vi "obj_DataLog Table Columns.vi"(0 "method":T7, 7 "tag":string, 9 "index":i32, 11 "error in (no error)":errorcluster, 12 "database":string, 13 "database infos":T8, 14 "table ref":refnum<vi>) -> (3 "column index":i32, 4 "#columns":i32, 6 "flag":bool, 8 "tag config":T2 {"logging parameters" format="%.2e"; "precision" items=["0", "1", "2", "3", "4", "5", "6", "7", "8", "9", "10", "11", "12", "13", "14", "15", "16", "17"]; "limit delay" format="%.2e"; "deadband" format="%.2e"}, 10 "mode":T1, 15 "error out":errorcluster)   [LabVIEW 2012]
doc: "Manages the addition, display, sorting, reordering, deletion, etc. of tags to/from the columns of the table control of the \"Log Table\" GUI."
uses:
  typedefs/t_Datalog Table Columns Methods.ctl
  typedefs/clusters/t_DataLog Tag Config.ctl
  typedefs/t_DataLog Temporal Types.ctl
  typedefs/t_DataLog Value Types.ctl
  typedefs/t_DataLog Numerical Format.ctl
  typedefs/t_DataLog Logging Algorithms.ctl
  typedefs/t_DataLog Table Retrieval Modes.ctl
  served/DataLog Database Infos_srv.ctl
  typedefs/t_DataLog Tag Info List Methods.ctl
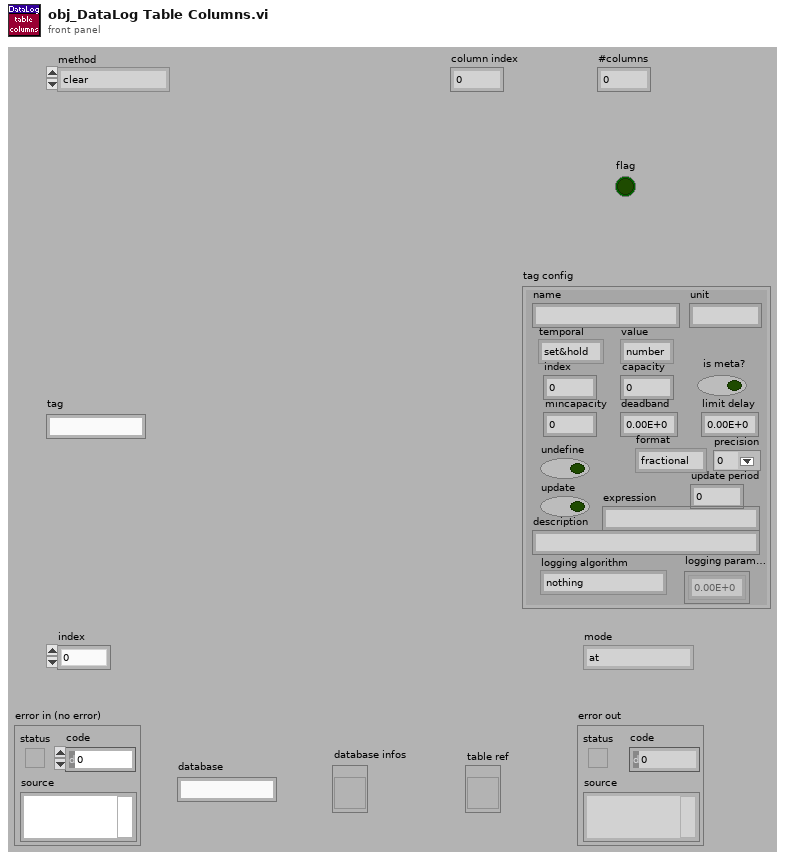
[diagram p1: front panel]
types:
  T1 = typedef "t_DataLog Table Retrieval Modes.ctl" = enum16{"at", "interpolate", "at+interpolate"}
  T2 = typedef "t_DataLog Tag Config.ctl" = cluster{"name":string, "unit":string, "temporal":T3, "value":T4, "index":i32, "capacity":i32, "is meta?":bool, "mincapacity":i32, "deadband":dbl, "limit delay":dbl, "format":T5, "precision":u8, "undefine":bool, "update":bool, "update period":u16, "expression":string, "description":string, "logging algorithm":T6, "logging parameters":dbl[]}
  T3 = typedef "t_DataLog Temporal Types.ctl" = enum16{"set&hold", "sample", "event"}
  T4 = typedef "t_DataLog Value Types.ctl" = enum16{"number", "string"}
  T5 = typedef "t_DataLog Numerical Format.ctl" = enum8{"fractional", "exponential", "engineering"}
  T6 = typedef "t_DataLog Logging Algorithms.ctl" = enum16{"nothing", "changes", "everything", "every Nth", "time threshold", "value threshold + prior", "t or v threshold", "t or v threshold + prior"}
  T7 = typedef "t_Datalog Table Columns Methods.ctl" = enum16{"clear", "#columns", "#number", "add", "insert", "remove", "change mode", "reorder", "sort", "index", "get by name", "interpolatable?", "ats?", "update"}
  T8 = typedef "DataLog Database Infos_srv.ctl" = refnum<vi>
  T9 = typedef "t_DataLog Tag Info List Methods.ctl" = enum16{"initialize", "create", "create empty", "rename", "delete", "test tag", "get", "get by name", "get default", "get list", "get path", "get subsets", "set subsets", "set config", "set capacity", "#tags", "go live", "set unlocked", "set mirrored"}
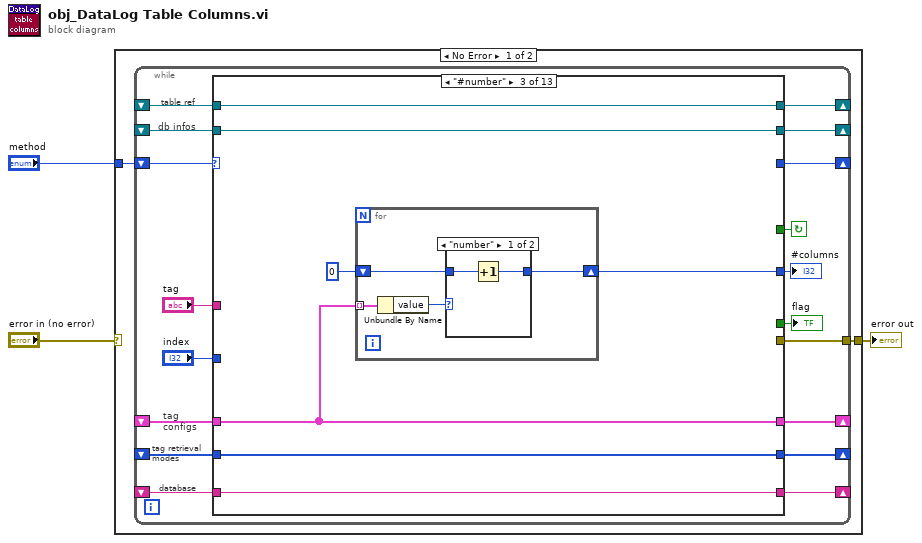
[diagram p0: block diagram]
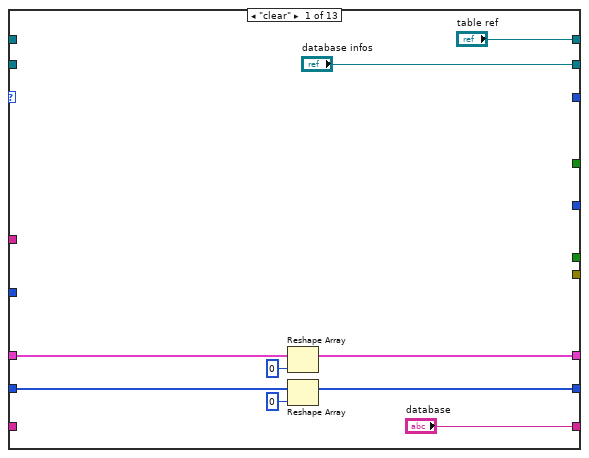
[diagram p2: hidden frame]
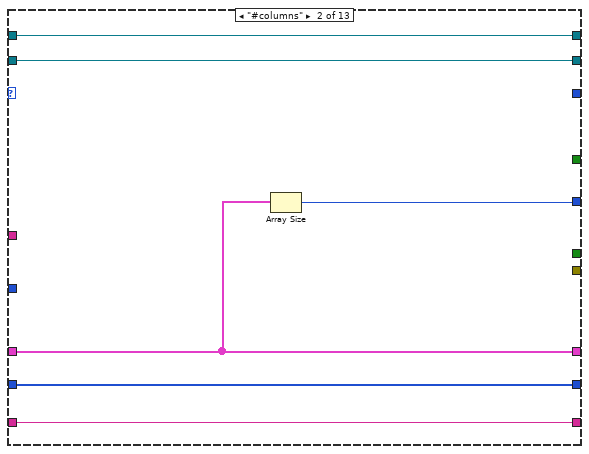
[diagram p3: hidden frame]
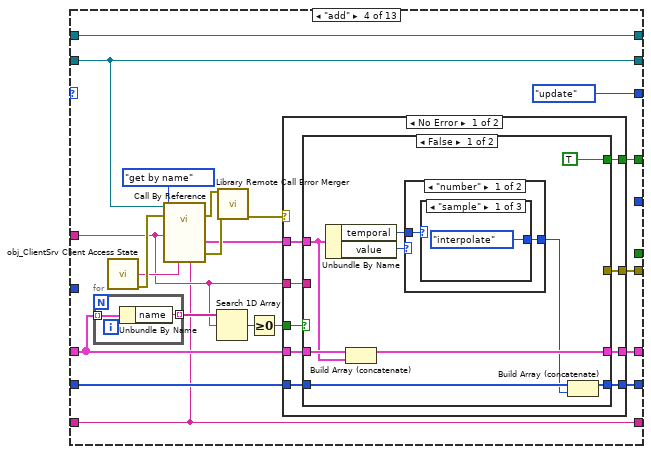
[diagram p5: hidden frame]
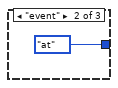
[diagram p6: hidden frame]
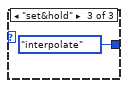
[diagram p7: hidden frame]
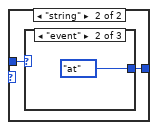
[diagram p8: hidden frame]
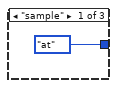
[diagram p9: hidden frame]
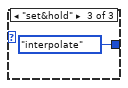
[diagram p10: hidden frame]
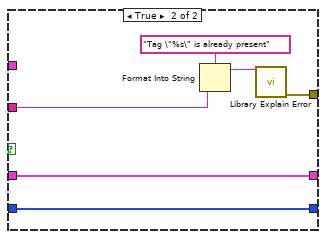
[diagram p11: hidden frame]
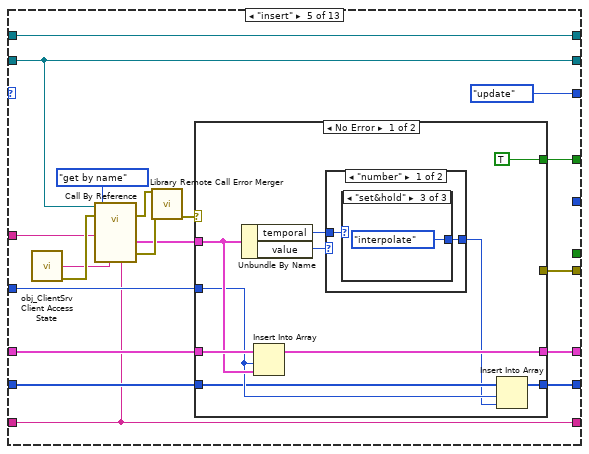
[diagram p13: hidden frame]
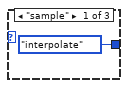
[diagram p14: hidden frame]
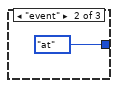
[diagram p15: hidden frame]
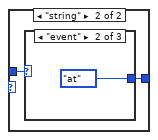
[diagram p16: hidden frame]
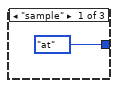
[diagram p17: hidden frame]
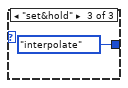
[diagram p18: hidden frame]
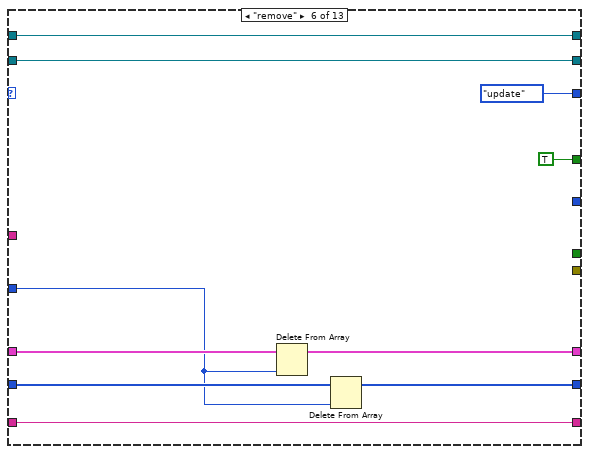
[diagram p20: hidden frame]
diagram:
  n1 = case shown="No Error" "error in (no error)" {
    selector: "error in (no error)" -> [_ w313]
    tunnel: [w4 w313] -> w2
    tunnel: "method" -> [w5 _]
    frame No Error {
      n2 = while {
        shift-right: [w23] -> _
        shift-left: _ -> [w22]
        shift-right: [w21] -> _
        shift-left: _ -> [w20]
        shift-right: [w19] -> _
        shift-left: _ -> [w18]
        shift-right: [w14] -> _
        shift-left: _ -> [w17]
        shift-right: [w15] -> _
        shift-left: _ -> [w16]
        shift-right: [w12] -> _
        shift-left: w5 -> [w13]
        tunnel: [w9] -> w4
        stop <- w11 continue-if-true
        # "tag retrieval\nmodes"
        # "tag\nconfigs"
        # "db infos"
        # "table ref"
        # "database"
        n3 = case shown="\"#number\"" w13 {
          selector: w13 -> [_ _ _ _ _ _ _ _ _ w232 _ _ _]
          tunnel: ["database infos" w36 w43 w59 w115 w162 w173 w190 w218 w237 w255 w278 w291] -> w23
          tunnel: w22 -> [_ w36 w43 w59 w115 w162 w173 w190 w218 w237 w255 w278 w291]
          tunnel: ["database" w37 w44 w53 w113 w164 w175 w191 w219 w238 w256 w279 w293] -> w21
          tunnel: w20 -> [_ w37 w44 w53 w113 w164 w175 w191 w219 w238 w256 w279 w293]
          tunnel: ["table ref" w35 w42 w73 w131 w163 w174 w189 w217 w236 w254 w277 w288] -> w19
          tunnel: w18 -> [_ w35 w42 w73 w131 w163 w174 w189 w217 w236 w254 w277 w288]
          tunnel: w17 -> [w29 w34 w41 w58 w123 w159 w170 w183 w213 w228 w252 w276 w292]
          tunnel: w16 -> [w26 w38 w45 w64 w120 w157 w168 w180 w220 w233 w253 w273 w294]
          tunnel: [w24 w38 w45 w63 w119 w156 w167 w181 w220 w233 w253 w273 w294] -> w15
          tunnel: [w27 w34 w41 w66 w122 w158 w170 w182 w212 w227 w252 w276 w292] -> w14
          tunnel: [_ _ _ t_Datalog_Table_Columns_Methods."update" ("method") t_Datalog_Table_Columns_Methods."update" ("method") t_Datalog_Table_Columns_Methods."update" ("method") t_Datalog_Table_Columns_Methods."update" ("method") t_Datalog_Table_Columns_Methods."update" ("method") t_Datalog_Table_Columns_Methods."update" ("method") _ _ _ _] -> w12
          tunnel: [_ _ _ w60 w116 TRUE TRUE w188 TRUE _ _ _ _] -> w11
          tunnel: "tag" -> [_ _ _ w54 w124 _ _ _ _ w231 _ _ _]
          tunnel: [_ _ _ w61 w117 _ _ _ _ _ _ _ w289] -> w9
          tunnel: "index" -> [_ _ _ _ w114 w155 w166 _ _ w230 w251 _ _]
          tunnel: [_ _ _ _ _ _ _ _ _ _ w249 w274 _] -> w7
          tunnel: [_ w33 w39 _ _ _ _ _ _ _ _ _ _] -> w6
          frame "clear" {
            n4 = Reshape Array(w29, 0 ("dimension size")) -> (w27:T2[])
            n5 = Reshape Array(w26, 0 ("dimension size")) -> (w24:T1[])
          }
          frame "#columns" {
            n6 = Array Size(array=w34) -> (size(s)=w33:i32)
          }
          frame "#number" {
            n7 = for {
              tunnel: w41 -> [w49] mode=indexing
              shift-right: [w47] -> w39
              shift-left: 0 -> [w46]
              n8 = Unbundle By Name(w49) -> ("value"=w48:T4)
              n9 = case shown="\"number\"" w48 {
                tunnel: [w51 w52] -> w47
                tunnel: w46 -> [w50 w52]
                frame "number" {
                  n10 = Increment(x=w50) -> (x+1=w51:i32)
                }
                frame "string" {
                }
              }
            }
          }
          frame "add" {
            n11 = for {
              tunnel: w58 -> [w75] mode=indexing
              tunnel: [w74] -> w57 mode=indexing
              n12 = Unbundle By Name(w75) -> ("name"=w74:string)
            }
            n13 = call "obj_ClientSrv Client Access State.vi"() -> ("certificate"=w69:string, "error out"=w71:errorcluster)  [unwired: 14 in]
            n14 = call-by-ref "?"(reference=w59, error in=w71, "method"=t_DataLog_Tag_Info_List_Methods."get by name", "tag or base tag"=w54, "certificate in"=w69, "database (current)"=w53) -> (error out=w72:errorcluster, "tag config out"=w65:T2, 15:"error out"=w70:errorcluster)  [unwired: 6 in, 5 out]
            n15 = Search 1D Array(1D array=w57, element=w54) -> (index of element=w56:i32)  [unwired: 1 in]
            n16 = call "Library Remote Call Error Merger.vi"("call by reference node error"=w72, "called VI error (no error)"=w70) -> ("error out"=w62:errorcluster)  [unwired: 13 in]
            n17 = Greater Or Equal To 0?(x=w56) -> (x >= 0?=w55:bool)
            n18 = case shown="No Error" w62 {
              selector: w62 -> [_ w112]
              tunnel: w58 -> [w84 w111]
              tunnel: [w83 w111] -> w66
              tunnel: w65 -> [w82 _]
              tunnel: w64 -> [w81 w110]
              tunnel: [w80 w110] -> w63
              tunnel: [w76 w112] -> w61
              tunnel: [w79 _] -> w60
              tunnel: w55 -> [w78 _]
              tunnel: w54 -> [w77 _]
              frame No Error {
                n19 = case shown="False" w78 {
                  tunnel: w84 -> [w93 w109]
                  tunnel: [w92 w109] -> w83
                  tunnel: w82 -> [w91 _]
                  tunnel: w81 -> [w88 w108]
                  tunnel: [w87 w108] -> w80
                  tunnel: [TRUE _] -> w79
                  tunnel: w77 -> [_ w104]
                  tunnel: [_ w107] -> w76
                  frame False {
                    n20 = Unbundle By Name(w91) -> ("temporal"=w90:T3, "value"=w89:T4)
                    n21 = Build Array (concatenate)(w93, w91) -> (w92:T2[])
                    n22 = case shown="\"number\"" w89 {
                      tunnel: w90 -> [w95 w100]
                      tunnel: [w94 w99] -> w86
                      frame "number" {
                        n23 = case shown="\"sample\"" w95 {
                          tunnel: [t_DataLog_Table_Retrieval_Modes."interpolate" ("retrieval modes") t_DataLog_Table_Retrieval_Modes."at" ("retrieval modes") t_DataLog_Table_Retrieval_Modes."interpolate" ("retrieval modes")] -> w94
                          frame "sample" {
                          }
                          frame "event" {
                          }
                          frame "set&hold" {
                          }
                        }
                      }
                      frame "string" {
                        n24 = case shown="\"event\"" w100 {
                          tunnel: [t_DataLog_Table_Retrieval_Modes."at" ("retrieval modes") t_DataLog_Table_Retrieval_Modes."at" ("retrieval modes") t_DataLog_Table_Retrieval_Modes."interpolate" ("retrieval modes")] -> w99
                          frame "sample" {
                          }
                          frame "event" {
                          }
                          frame "set&hold" {
                          }
                        }
                      }
                    }
                    n25 = Build Array (concatenate)(w88, w86) -> (w87:T1[])
                  }
                  frame True {
                    n26 = Format Into String(format string="Tag \"%s\" is already present", w104) -> (resulting string=w106:string)  [unwired: 2 in, 1 out]
                    n27 = call "Library Explain Error.vi"("explanation prefix (none)"=w106) -> ("explained error"=w107:errorcluster)  [unwired: 14 in]
                  }
                }
              }
              frame Error {
              }
            }
          }
          frame "insert" {
            n28 = call "obj_ClientSrv Client Access State.vi"() -> ("certificate"=w127:string, "error out"=w129:errorcluster)  [unwired: 14 in]
            n29 = call-by-ref "?"(reference=w115, error in=w129, "method"=t_DataLog_Tag_Info_List_Methods."get by name", "tag or base tag"=w124, "certificate in"=w127, "database (current)"=w113) -> (error out=w130:errorcluster, "tag config out"=w121:T2, 15:"error out"=w128:errorcluster)  [unwired: 6 in, 5 out]
            n30 = call "Library Remote Call Error Merger.vi"("call by reference node error"=w130, "called VI error (no error)"=w128) -> ("error out"=w118:errorcluster)  [unwired: 13 in]
            n31 = case shown="No Error" w118 {
              selector: w118 -> [_ w154]
              tunnel: w123 -> [w141 w153]
              tunnel: [w140 w153] -> w122
              tunnel: w121 -> [w136 _]
              tunnel: w120 -> [w134 w152]
              tunnel: [w133 w152] -> w119
              tunnel: [_ w154] -> w117
              tunnel: [TRUE _] -> w116
              tunnel: w114 -> [w135 _]
              frame No Error {
                n32 = Unbundle By Name(w136) -> ("temporal"=w139:T3, "value"=w138:T4)
                n33 = Insert Into Array(array=w141, index=w135, new element=w136) -> (w140:T2[])
                n34 = case shown="\"number\"" w138 {
                  tunnel: w139 -> [w143 w148]
                  tunnel: [w142 w147] -> w132
                  frame "number" {
                    n35 = case shown="\"set&hold\"" w143 {
                      tunnel: [t_DataLog_Table_Retrieval_Modes."interpolate" ("retrieval modes") t_DataLog_Table_Retrieval_Modes."at" ("retrieval modes") t_DataLog_Table_Retrieval_Modes."interpolate" ("retrieval modes")] -> w142
                      frame "sample" {
                      }
                      frame "event" {
                      }
                      frame "set&hold" {
                      }
                    }
                  }
                  frame "string" {
                    n36 = case shown="\"event\"" w148 {
                      tunnel: [t_DataLog_Table_Retrieval_Modes."at" ("retrieval modes") t_DataLog_Table_Retrieval_Modes."at" ("retrieval modes") t_DataLog_Table_Retrieval_Modes."interpolate" ("retrieval modes")] -> w147
                      frame "sample" {
                      }
                      frame "event" {
                      }
                      frame "set&hold" {
                      }
                    }
                  }
                }
                n37 = Insert Into Array(array=w134, index=w135, new element=w132) -> (w133:T1[])
              }
              frame Error {
              }
            }
          }
          frame "remove" {
            n38 = Delete From Array(array=w159, index=w155) -> (array with subset deleted=w158:T2[])  [unwired: 1 in, 1 out]
            n39 = Delete From Array(array=w157, index=w155) -> (array with subset deleted=w156:T1[])  [unwired: 1 in, 1 out]
          }
          frame "change mode" {
            n40 = Index Array(array=w168, index=w166) -> (element=w169:T1)
            n41 = case shown="\"at\"" w169 {
              tunnel: [t_DataLog_Table_Retrieval_Modes."at+interpolate" ("retrieval modes") t_DataLog_Table_Retrieval_Modes."at" ("retrieval modes") t_DataLog_Table_Retrieval_Modes."interpolate" ("retrieval modes")] -> w165
              frame "interpolate" {
              }
              frame "at+interpolate" {
              }
              frame "at" {
              }
            }
            n42 = Replace Array Subset(array=w168, new element=w165, index=w166) -> (w167:T1[])
          }
          frame "reorder" {
            n43 = for {
              tunnel: w183 -> [w209] mode=indexing
              tunnel: [w208] -> w184 mode=indexing
              n44 = Unbundle By Name(w209) -> ("name"=w208:string)
            }
            n45 = call "ui_DataLog Reorder Listed Strings.vi"("prompt"="Reorder tag columns:", "list of strings"=w184) -> ("OKed?"=w186:bool, "reordered strings"=w185:string[])  [unwired: 12 in]
            n46 = case shown="True" w186 {
              tunnel: [_ TRUE] -> w188
              tunnel: w185 -> [_ w199]
              tunnel: w184 -> [_ w198]
              tunnel: w183 -> [w193 w197]
              tunnel: [w193 w196] -> w182
              tunnel: [w192 w195] -> w181
              tunnel: w180 -> [w192 w194]
              frame False {
              }
              frame True {
                n47 = for {
                  tunnel: w199 -> [w206] mode=indexing
                  tunnel: w198 -> [w207]
                  tunnel: w197 -> [w205]
                  tunnel: [w204] -> w196 mode=indexing
                  tunnel: [w203] -> w195 mode=indexing
                  tunnel: w194 -> [w202]
                  n48 = Search 1D Array(1D array=w207, element=w206) -> (index of element=w201:i32)  [unwired: 1 in]
                  n49 = Index Array(array=w205, index=w201) -> (element=w204:T2)
                  n50 = Index Array(array=w202, index=w201) -> (element=w203:T1)
                }
              }
            }
          }
          frame "sort" {
            # "avoid LV7 bug"
            n51 = for "prepend for sorting" {
              tunnel: w213 -> [w224] mode=indexing
              tunnel: [w226] -> w215 mode=indexing
              # "Lower case. This makes\nthe sort case insensitive\nand gives the underscore\na lower priority so that\nmeta tags group with\ntheir base tag."
              n52 = Unbundle By Name(w224) -> ("name"=w223:string)
              n53 = To Lower Case(string=w223) -> (all lower case string=w225:string)
              n54 = Bundle(w225, "tag config out"=w224) -> (w226:cluster{string, "tag config out":T2})  [unwired: 1 in]
            }
            n55 = Sort 1D Array(array=w215) -> (sorted array=w216:cluster{string, "tag config out":T2}[])
            n56 = Sort 1D Array(array=w216) -> (sorted array=w214:cluster{string, "tag config out":T2}[])
            n57 = for {
              tunnel: w214 -> [w222] mode=indexing
              tunnel: [w221] -> w212 mode=indexing
              n58 = Unbundle(w222) -> ("tag config out"=w221:T2)  [unwired: 1 out]
            }
          }
          frame "index", "get by name" {
            n59 = case shown="\"get by name\"" w232 {
              tunnel: w231 -> [_ _ w244]
              tunnel: w230 -> [w240 w242 _]
              tunnel: [w240 w242 w243] -> w229
              tunnel: w228 -> [w239 w241 w246]
              tunnel: [w239 w241 w246] -> w227
              frame Default {
              }
              frame "index" {
              }
              frame "get by name" {
                n60 = for {
                  tunnel: w246 -> [w248] mode=indexing
                  tunnel: [w247] -> w245 mode=indexing
                  n61 = Unbundle By Name(w248) -> ("name"=w247:string)
                }
                n62 = Search 1D Array(1D array=w245, element=w244) -> (index of element=w243:i32)  [unwired: 1 in]
                "column index" <- w243
              }
            }
            n63 = Index Array(array=w227, index=w229) -> (element=→"tag config":T2)
            n64 = Index Array(array=w233, index=w229) -> (element=→"mode":T1)
          }
          frame "interpolatable?" {
            n65 = Greater Or Equal To 0?(x=w251) -> (x >= 0?=w250:bool)
            n66 = case shown="True" w250 {
              tunnel: w252 -> [_ w259]
              tunnel: [_ w258] -> w249
              tunnel: w251 -> [_ w257]
              frame False {
              }
              frame True {
                n67 = Index Array(array=w259, index=w257) -> (element=w260:T2)
                n68 = Unbundle By Name(w260) -> ("temporal"=w262:T3, "value"=w261:T4)
                n69 = case shown="\"number\"" w261 {
                  tunnel: w262 -> [w264 w269]
                  tunnel: [w263 w268] -> w258
                  frame "number" {
                    n70 = case shown="\"set&hold\"" w264 {
                      tunnel: [TRUE FALSE TRUE] -> w263
                      frame "sample" {
                      }
                      frame "event" {
                      }
                      frame "set&hold" {
                      }
                    }
                  }
                  frame "string" {
                    n71 = case shown="\"event\"" w269 {
                      tunnel: [FALSE FALSE TRUE] -> w268
                      frame "sample" {
                      }
                      frame "event" {
                      }
                      frame "set&hold" {
                      }
                    }
                  }
                }
              }
            }
          }
          frame "ats?" {
            n72 = for {
              shift-right: [w280] -> w274
              shift-left: FALSE -> [w281]
              tunnel: w273 -> [w282] mode=indexing
              n73 = case shown="\"at\", \"at+interpolate\"" w282 {
                tunnel: w281 -> [_ w284]
                tunnel: [TRUE w284] -> w280
                frame "at", "at+interpolate" {
                }
                frame "interpolate" {
                }
              }
            }
          }
          frame "update" {
            n74 = for {
              tunnel: w292 -> [w311] mode=indexing
              tunnel: [w308] -> w290 mode=indexing
              tunnel: w294 -> [w307] mode=indexing
              tunnel: [" "] -> w287 mode=indexing
              w312 = "\n"
              n75 = Unbundle By Name(w311) -> ("temporal"=w305:T3, "value"=w304:T4, "name"=w310:string, "unit"=w309:string, "logging algorithm"=w300:T6)
              n76 = Format Into String(w307) -> (resulting string=w303:string)  [unwired: 3 in, 1 out]
              n77 = Equal?(x=w300, y=t_DataLog_Logging_Algorithms."nothing" ("logging algorithm")) -> (x = y?=w298:bool)
              n78 = Format Into String(format string="%s/%s", w305, w304) -> (resulting string=w302:string)  [unwired: 2 in, 1 out]
              n79 = Select(t="!", s=w298, f="") -> (s? t:f=w295:string)
              n80 = Concatenate Strings(w310, w312, w309, w312, w295, w302, w312, w303, w312) -> (w308:string)
            }
            n81 = Build Array(w287) -> (w286:string[][])
            n82 = property class="Tbl"(reference=w288, "Column Header Strings[]"=w290, "Value"=w286, "Row Header Strings[]"=string[] [] ("Row Headers[]")) -> (error out=w289:errorcluster)  [unwired: 1 in, 1 out]
          }
        }
        "flag" <- w7
        "#columns" <- w6
      }
    }
    frame Error {
    }
  }
  "error out" <- w2
